vi "SingleChannelCode_NI9219.vi"() -> ()   [LabVIEW 2022 SP3]
uses:
  <vilib>/DAQmx/read.llb/DAQmx Read (Analog Wfm 1Chan NSamp).vi
  <vilib>/Analysis/baseanly.llb/Mean (DBL).vi
  <vilib>/DAQmx/create/channels.llb/DAQmx Create Channel (AI-Voltage-Basic).vi
  <vilib>/DAQmx/configure/timing.llb/DAQmx Timing (Sample Clock).vi
  <vilib>/DAQmx/miscellaneous.llb/DAQmx Fill In Error Info.vi
  <resource>/objmgr/daqmx.rc
  <vilib>/Analysis/NI_AALBase.lvlib
panel:
  out "mean":dbl format="%0.2f"
  out "AI.Min":dbl
  out "AI.Max":dbl
  in  "error in":errorcluster
  in  "task in":refnum<k21>
  out "New Calibration":dbl[](graph)
  out "Voltage Signal":dbl[](graph)
  out "Arbitrary Calibration":dbl[](graph)
  out "Read Rate":dbl
  out "SampClk.Rate":dbl
  out "relative seconds":dbl format="%_19f"
  out "error out 2":errorcluster
  in  "stop":bool
  out "Chamber Pressure":waveform(dbl)(graph)
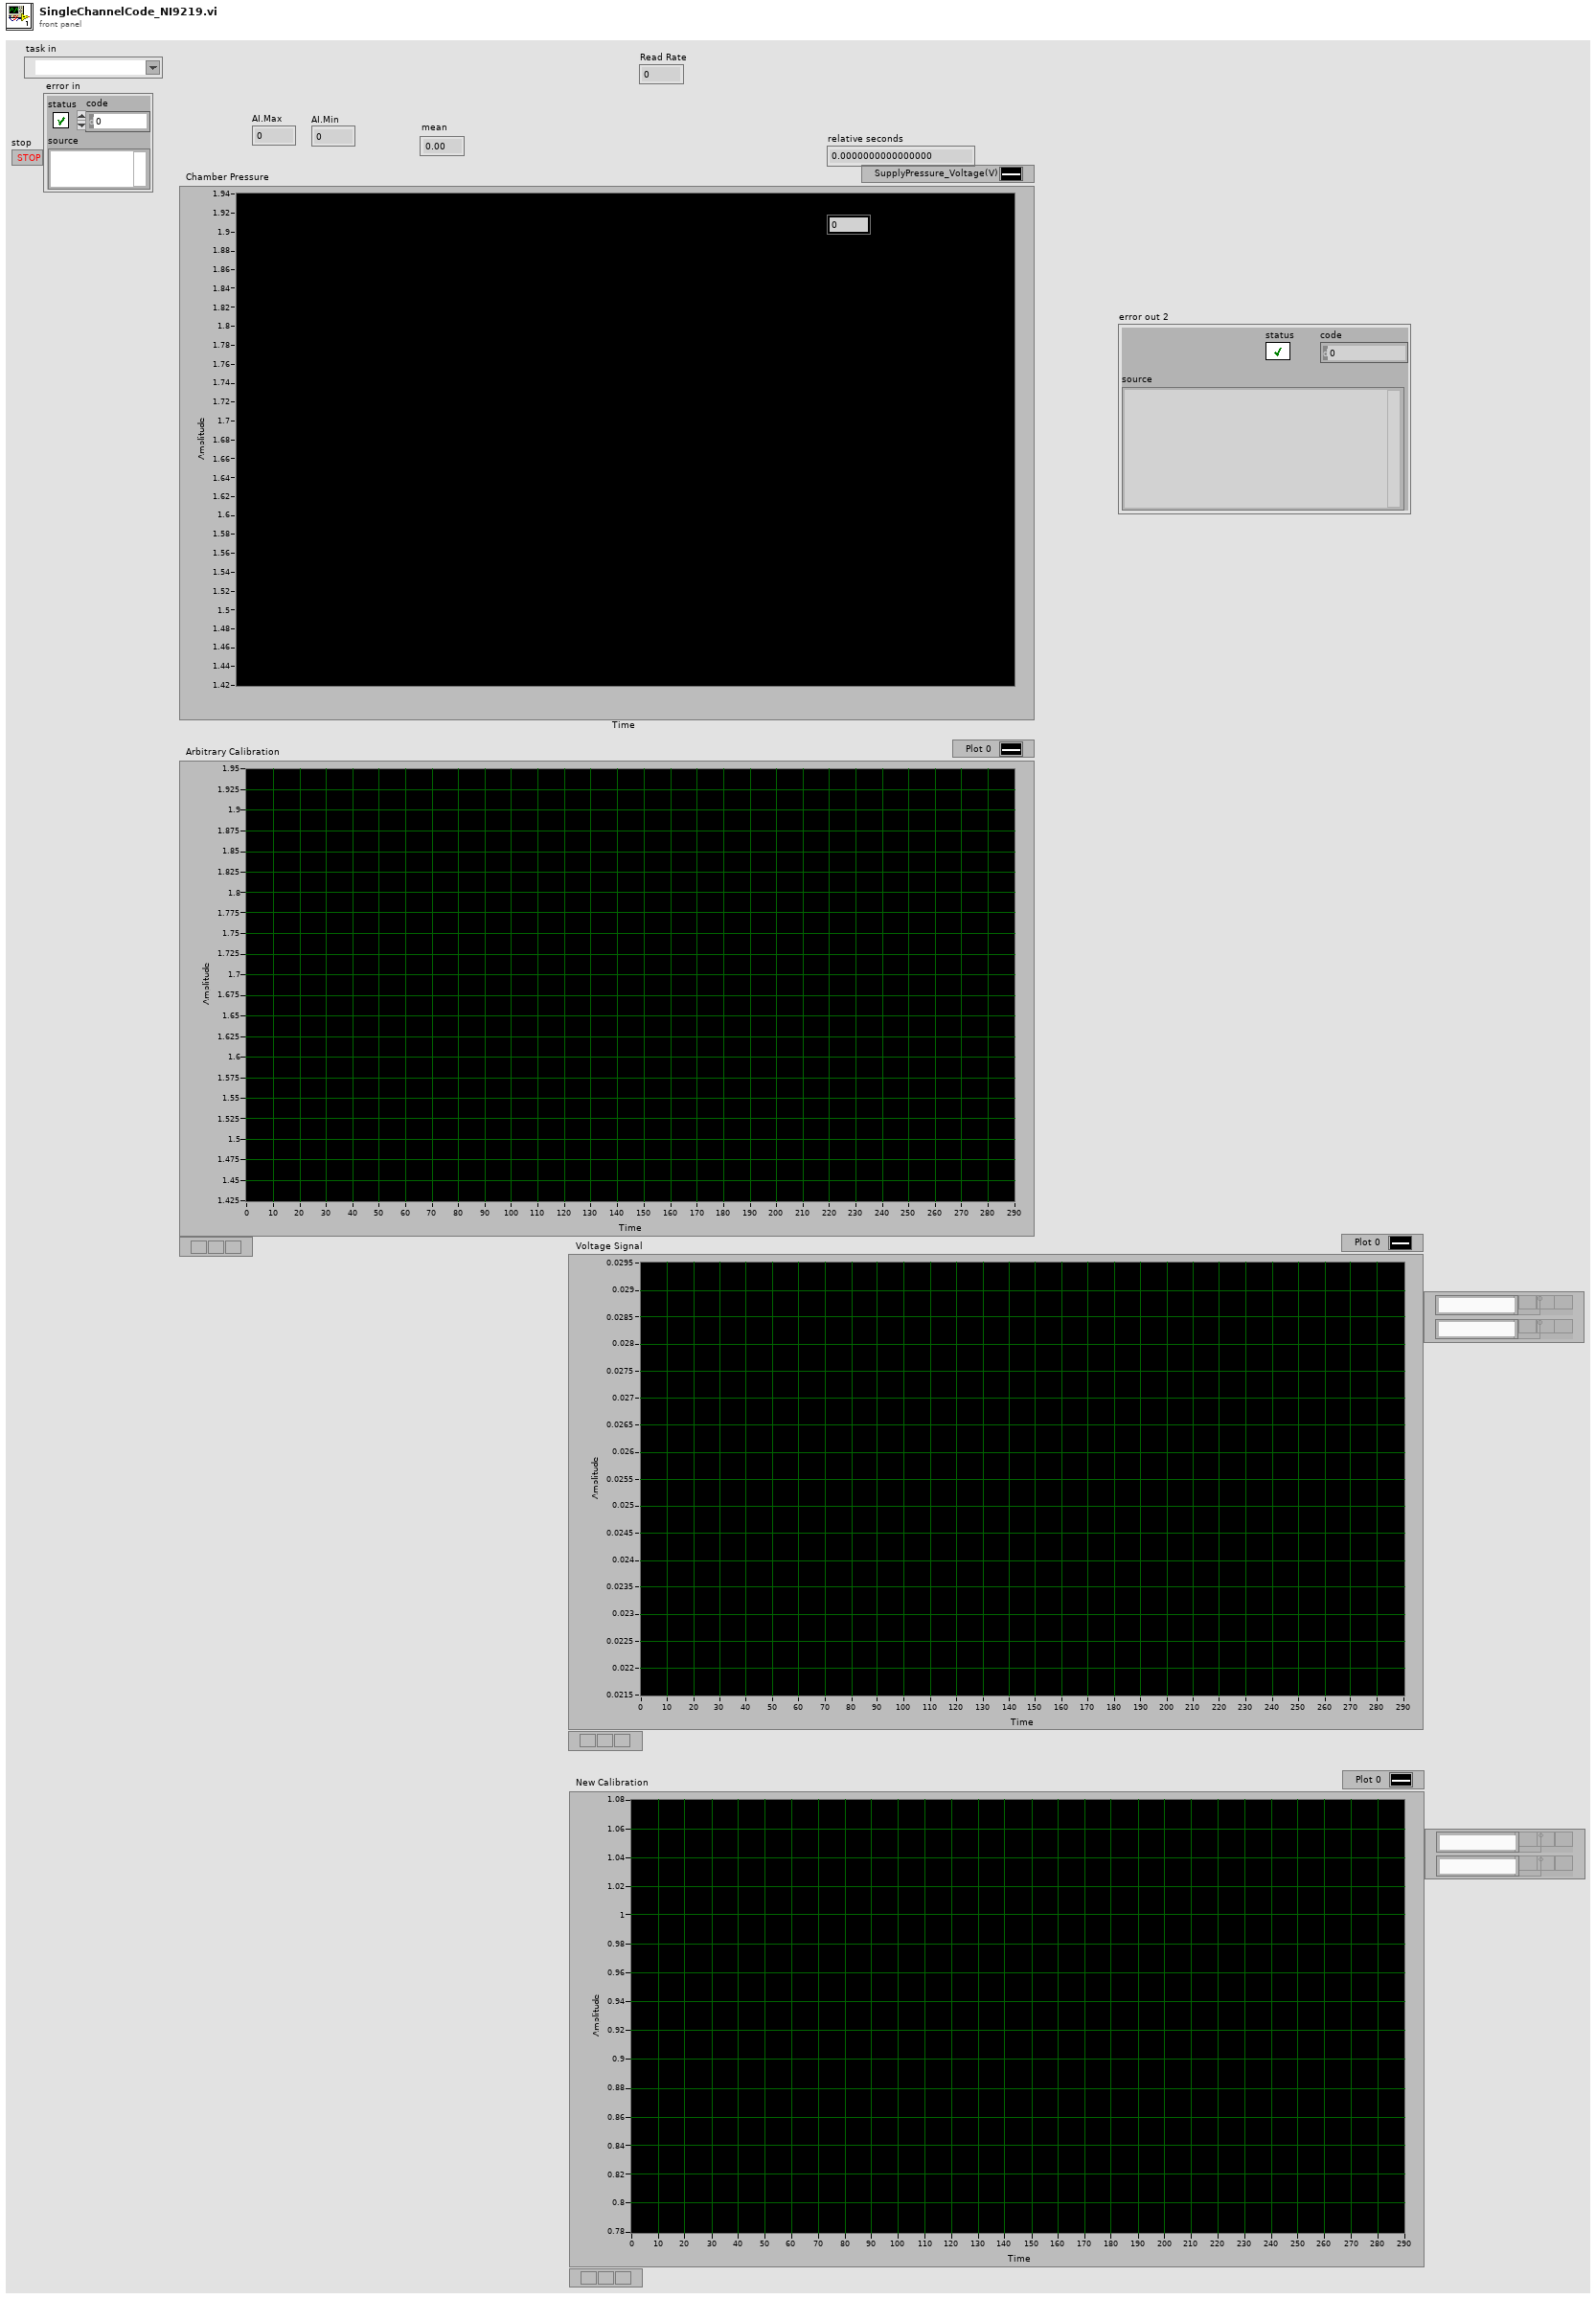
[diagram p1: front panel]
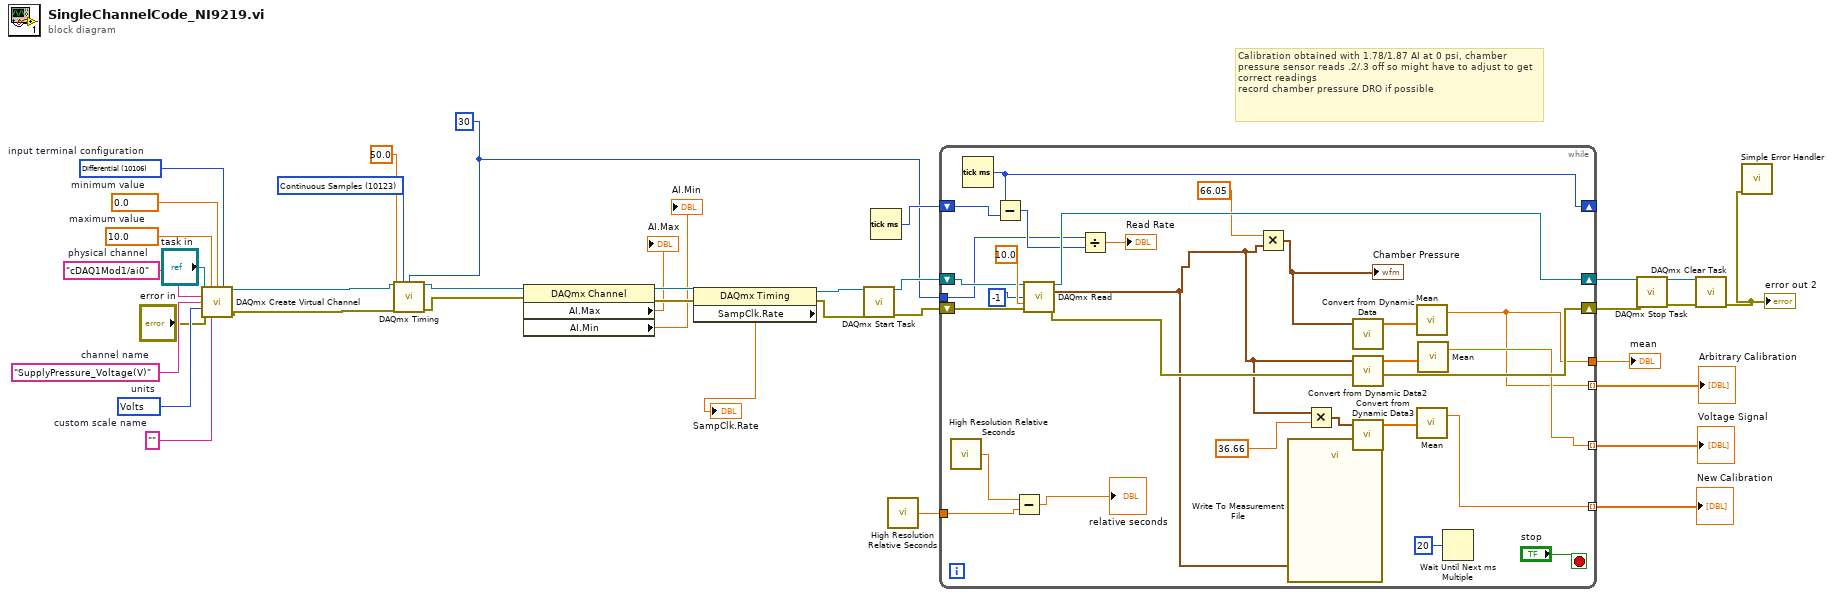
[diagram p0: block diagram]
diagram:
  w12 = 10106 items=["default"=-1, "RSE"=10083, "NRSE"=10078, "Differential"=10106, "Pseudodifferential"=12529]  # input terminal configuration
  w13 = 10348 items=["Volts"=10348, "From Custom Scale"=10065]  # units
  w14 = "SupplyPressure_Voltage(V)"  # channel name
  w15 = ""  # custom scale name
  w16 = 0.0  # minimum value
  w17 = 10.0  # maximum value
  w18 = "cDAQ1Mod1/ai0"  # physical channel
  w28 = 10123 items=["Finite Samples"=10178, "Continuous Samples"=10123, "Hardware Timed Single Point"=12522] ("sample mode")
  w26 = 30 ("samples per channel")
  # "Calibration obtained with 1.78/1.87 AI at 0 psi, chamber pressure sensor reads .2/.3 off so might have to adjust to get correct readings\nrecord chamber pressure DRO if possible"
  n1 = call-poly <vilib>:"DAQmx Create Virtual Channel.vi"("task in"="task in", "maximum value"=w17, "minimum value"=w16, "input terminal configuration"=w12, "physical channels"=w18, "name to assign"=w14, "units"=w13, "error in"="error in", "custom scale name"=w15) -> ("task out"=w9:refnum<k21>, "error out"=w8:errorcluster)  [unwired: 5 in]
  n2 = call-poly <vilib>:"DAQmx Timing.vi"("task/channels in"=w9, "sample mode"=w28, "samples per channel"=w26, "rate"=50.0, "error in"=w8) -> ("task out"=w2:refnum<k21>, "error out"=w1:errorcluster)  [unwired: 9 in]
  n3 = property class="DAQmx Channel"(reference=w2, error in=w1) -> (reference out=w7:refnum<k21>, error out=w6:errorcluster, "AI.Max"=→"AI.Max":dbl, "AI.Min"=→"AI.Min":dbl)
  n4 = property class="DAQmx Timing"(reference=w7, error in=w6) -> (reference out=w25:refnum<k21>, error out=w24:errorcluster, "SampClk.Rate"=→"SampClk.Rate":dbl)
  n5 = call <vilib>:"DAQmx Start Task.vi"("task/channels in"=w25, "error in"=w24) -> ("task out"=w30:refnum<k21>, "error out"=w29:errorcluster)  [unwired: 12 in]
  n6 = Tick Count (ms)() -> (millisecond timer value=w27:u32)
  n7 = call <vilib>:"High Resolution Relative Seconds.vi"() -> ("relative seconds"=w23:dbl)
  n8 = while {
    shift-right: [w60] -> w36
    shift-left: w30 -> [w62]
    shift-right: [w59] -> w35
    shift-left: w29 -> [w61]
    shift-right: [w56] -> _
    shift-left: w27 -> [w57]
    tunnel: w26 -> [w52]
    tunnel: w23 -> [w50]
    tunnel: [w39] -> w22 mode=indexing
    tunnel: [w44] -> w21 mode=indexing
    tunnel: [w40] -> w20 mode=indexing
    tunnel: [w39] -> w3
    stop <- "stop" stop-if-true
    n9 = call <vilib>:"High Resolution Relative Seconds.vi"() -> ("relative seconds"=w51:dbl)
    n10 = Tick Count (ms)() -> (millisecond timer value=w56:u32)
    n11 = Subtract(x=w56, y=w57) -> (x-y=w55:u32)
    n12 = Subtract(x=w51, y=w50) -> (x-y=→"relative seconds":dbl)
    n13 = call-poly <vilib>:"DAQmx Read.vi"("task/channels in"=w62, "number of samples per channel"=-1, "timeout"=10.0, "error in"=w61) -> ("task out"=w60:refnum<k21>, "data"=w38:waveform(dbl), "error out"=w59:errorcluster)  [unwired: 9 in]
    n14 = Divide(x=w52, y=w55) -> (x/y=→"Read Rate":dbl)
    n15 = Multiply(x=66.05, y=w38) -> (x*y=w46:waveform(dbl))
    "Chamber Pressure" <- w46
    n16 = call "Write To Measurement File"("Signals"=w38) -> ()  [unwired: 16 in, 3 out]
    n17 = Multiply(x=w38, y=36.66) -> (x*y=w41:waveform(dbl))
    n18 = call "Convert from Dynamic Data"("Dynamic Data Type"=w46) -> ("Array"=w47:dbl[])  [unwired: 3 in]
    n19 = call "Convert from Dynamic Data2"("Dynamic Data Type"=w38) -> ("Array"=w45:dbl[])  [unwired: 3 in]
    n20 = call "Convert from Dynamic Data3"("Dynamic Data Type"=w41) -> ("Array"=w43:dbl[])  [unwired: 3 in]
    n21 = call-poly <vilib>:"Mean.vi"("X"=w47) -> ("mean"=w39:dbl)  [unwired: 1 out]
    n22 = call-poly <vilib>:"Mean.vi"("X"=w43) -> ("mean"=w40:dbl)  [unwired: 1 out]
    n23 = call-poly <vilib>:"Mean.vi"("X"=w45) -> ("mean"=w44:dbl)  [unwired: 1 out]
    n24 = Wait Until Next ms Multiple(millisecond multiple=u32 20) -> ()  [unwired: 1 out]
  }
  "Arbitrary Calibration" <- w22
  "Voltage Signal" <- w21
  "New Calibration" <- w20
  "mean" <- w3
  n25 = call <vilib>:"DAQmx Stop Task.vi"("task/channels in"=w36, "error in"=w35) -> ("task out"=w34:refnum<k21>, "error out"=w33:errorcluster)  [unwired: 12 in]
  n26 = call <vilib>:"DAQmx Clear Task.vi"("task in"=w34, "error in"=w33) -> ("error out"=w19:errorcluster)  [unwired: 13 in]
  "error out 2" <- w19
  n27 = call <vilib>:"Simple Error Handler.vi"("error in (no error)"=w19) -> ()  [unwired: 4 in, 5 out]
